vi "Auto Configuration.vi"() -> ()   [LabVIEW 2017]
uses:
  2018_Trobots_5013_Robot/Support Code/Blocks.ctl
  2018_Trobots_5013_Robot/Support Code/Routines.ctl
  2018_Trobots_5013_Robot/Auto Code/Block Clusters/Far--L.ctl
  2018_Trobots_5013_Robot/Auto Code/Block Clusters/end Sw--sq C1.ctl
  2018_Trobots_5013_Robot/Auto Code/Block Clusters/end cube--C1.ctl
  2018_Trobots_5013_Robot/Auto Code/Block Clusters/C1--d Hi.ctl
  2018_Trobots_5013_Robot/Auto Code/Block Clusters/C1--C3.ctl
  2018_Trobots_5013_Robot/Auto Code/Block Clusters/C3--C4.ctl
  2018_Trobots_5013_Robot/Auto Code/Block Clusters/d Hi--C1.ctl
  2018_Trobots_5013_Robot/Auto Code/Block Clusters/C3--End Sw.ctl
  2018_Trobots_5013_Robot/Auto Code/Block Clusters/C3--cube Sw.ctl
  2018_Trobots_5013_Robot/Auto Code/Block Clusters/M--front RSw.ctl
  2018_Trobots_5013_Robot/Auto Code/Block Clusters/L--C1.ctl
  2018_Trobots_5013_Robot/Auto Code/Block Clusters/C1--end cube.ctl
  2018_Trobots_5013_Robot/Auto Code/Block Clusters/L--end Sw.ctl
  2018_Trobots_5013_Robot/Auto Code/Block Clusters/front Sw--L.ctl
  2018_Trobots_5013_Robot/Auto Code/Block Clusters/M--front LSw.ctl
  2018_Trobots_5013_Robot/Auto Code/Block Clusters/SQ Hi--C1.ctl
  2018_Trobots_5013_Robot/Auto Code/Block Clusters/C1--sq Hi.ctl
  2018_Trobots_5013_Robot/Auto Code/Block Clusters/front Sw--P cube1.ctl
  2018_Trobots_5013_Robot/Auto Code/Block Clusters/P cube1--front Sw.ctl
  Routines and Block Data.ctl
  <vilib>/Rock Robotics/Network Tables/NT Write Boolean.vi
panel:
  in  "Reposition":bool
  out "appended path":path=path "C:/Program Files (x86)/FRC Dashboard/data/C1--end cube.jpg"
  out "Tab Control":T1(tab)=enum."2"
  in  "Far--L":T2={"1a"=0.0, "1d"=100.5, "1s"=0.8}
  in  "L--end Sw":T3={"1d"=48.0, "1s"=0.8, "2t"=3.0, "3a"=90.0, "4d"=21.5, "4s"=0.8}
  in  "end Sw--sq C1":T4={"1a"=-90.0, "1d"=-48.0, "1s"=-0.65, "2d"=67.25, "2s"=0.75}
  in  "end cube--C1":T5={"1a"=124.0, "1d"=0.0, "1s"=0.0, "2a"=0.0}
  in  "C1--d Hi":T6={"1t"=6.5, "2d"=55.0, "2s"=0.65, "3a"=38.0, "4d"=10.0, "4s"=0.5}
  in  "C1--C3":T7={"1a"=90.0, "2d"=185.0, "2s"=1.0}
  in  "C3 to C4":T8
  in  "d Hi--C1":T9={"1a"=38.0, "1d"=18.0, "1s"=0.8, "3t"=0.0, "4d"=33.0, "4s"=1.0}
  in  "C3--End Sw":T10={"1a"=90.0, "1d"=45.31, "1s"=0.8, "2a"=180.0, "3t"=3.0, "4d"=67.25, "4s"=0.7, "5a"=-90.0, "6d"=19.31, "6s"=0.5}
  in  "C3--cube Sw":T11
  in  "M--front LSw":T12={"1d"=14.0, "1s"=1.0, "2a"=-51.5, "3t"=3.0, "4d"=141.0, "4s"=1.0, "5a"=0.0, "6d"=19.5, "6s"=0.5}
  in  "M--front RSw":T13
  in  "front Sw--L":T14={"1d"=14.0, "1s"=-1.0, "2a"=90.0, "3t"=0.0, "4d"=58.25, "4s"=1.0, "5a"=0.0}
  in  "L--C1":T15={"1a"=0.0, "1d"=115.25, "1s"=0.8}
  in  "C1--end cube":T16={"1a"=124.0, "2d"=28.0, "2s"=0.65, "3g"=10.0, "4t"=1.0}
  in  "sq Hi--C1":T17
  in  "C1--sq Hi":T18
  in  "front Sw--P cube1":T19
  in  "P cube1--front Sw":T20={"1a"=0.0, "1d"=40.0, "1s"=-0.85, "2a"=-90.0, "1t"=3.0, "2d"=57.0, "2s"=1.0, "3d"=81.0, "3s"=0.65}
  in  "Remove":bool
  in  "Index":i32=1 min=1 step=1
  in  "Insert":bool
  in  "Routines":T21
  in  "Routine Blocks":T22[](array[typedef])=[enum."M--front LSw", enum."front Sw--L", enum."L--C1", enum."C1--end cube", enum."end cube--C1", enum."C1--d Hi", enum."", enum."", enum."", enum."", enum."", enum."", enum."", enum."", enum."", enum."", enum."", enum."", enum."", enum."", enum."", enum."", enum."", enum."", enum."", enum."", enum.""]
  in  "Cancel":bool
  in  "Done":bool
  in  "Block to Modify":T22=enum."Far--L"
  out "block picture":picture
  # "1"
  # "2"
  # "3"
  # "4"
  # "5"
  # "6"
  # "7"
  # "8"
  # "9"
  # "10"
  # "11"
  # "12"
  # "13"
  # "14"
  # "15"
  # "16"
  # "17"
  # "18"
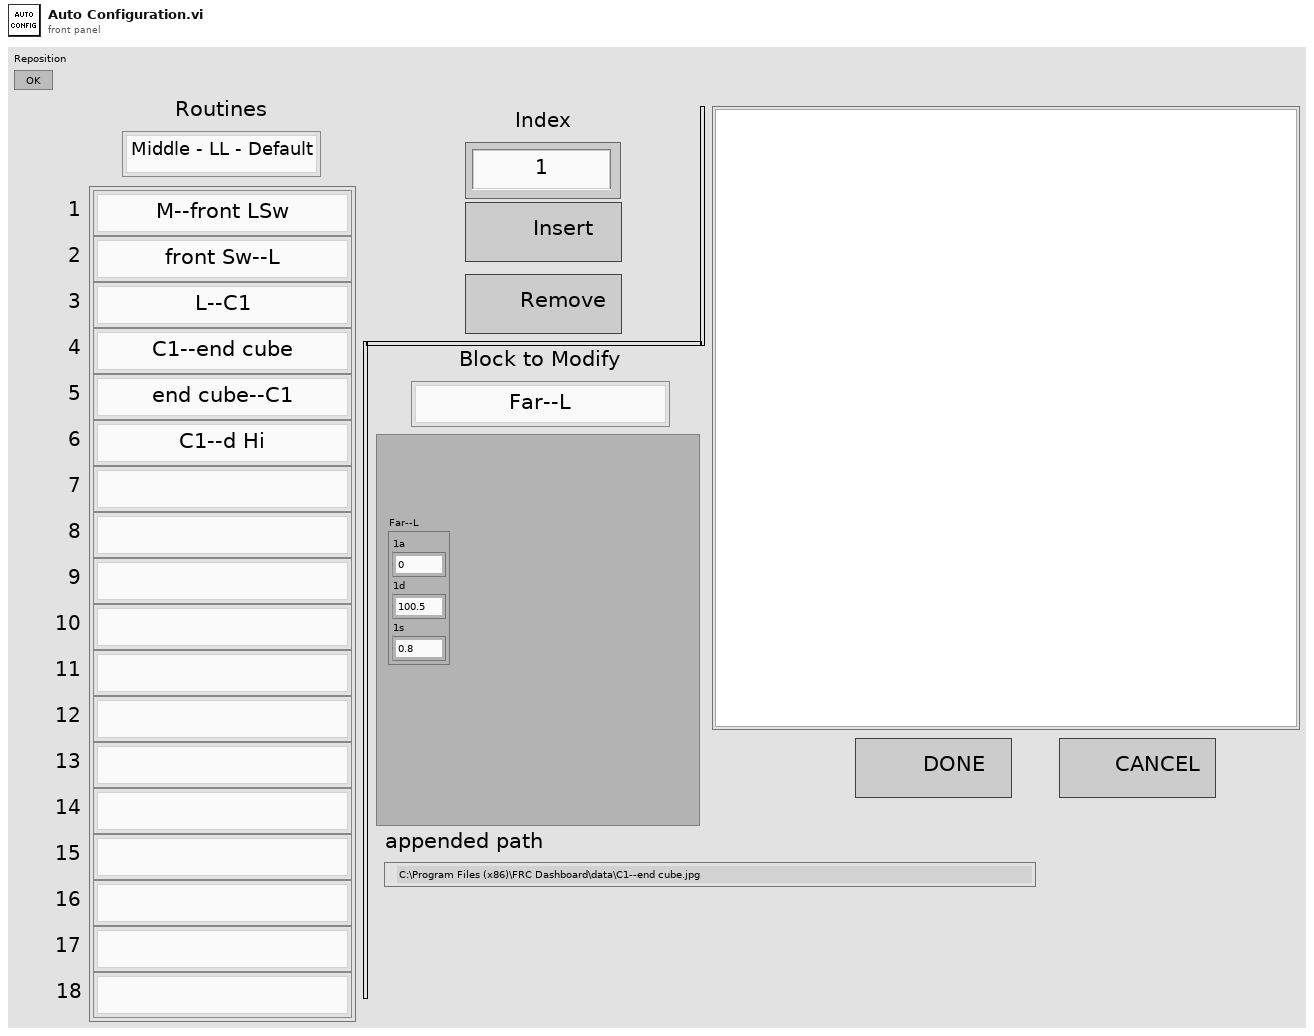
[diagram p1: front panel]
types:
  T1 = enum32{"0", "1", "2", "3", "4", "5", "6", "7", "8", "9", "9 2", "9 3", "9 4", "9 5", "front Sw--L", "L--C1", "C1--end cube", "C1--end cube 2", "C1--end cube 3", "C1--end cube 4", "C1--end cube 5"}
  T2 = typedef "Far--L.ctl" = cluster{"1a":dbl, "1d":dbl, "1s":dbl}
  T3 = typedef "L--end Sw.ctl" = cluster{"1d":dbl, "1s":dbl, "2t":dbl, "3a":dbl, "4d":dbl, "4s":dbl}
  T4 = typedef "end Sw--sq C1.ctl" = cluster{"1a":dbl, "1d":dbl, "1s":dbl, "2d":dbl, "2s":dbl}
  T5 = typedef "end cube--C1.ctl" = cluster{"1a":dbl, "1d":dbl, "1s":dbl, "2a":dbl}
  T6 = typedef "C1--d Hi.ctl" = cluster{"1t":dbl, "2d":dbl, "2s":dbl, "3a":dbl, "4d":dbl, "4s":dbl}
  T7 = typedef "C1--C3.ctl" = cluster{"1a":dbl, "2d":dbl, "2s":dbl}
  T8 = typedef "C3--C4.ctl" = cluster{"1a":dbl, "1d":dbl, "1s":dbl}
  T9 = typedef "d Hi--C1.ctl" = cluster{"1a":dbl, "1d":dbl, "1s":dbl, "3t":dbl, "4d":dbl, "4s":dbl}
  T10 = typedef "C3--End Sw.ctl" = cluster{"1a":dbl, "1d":dbl, "1s":dbl, "2a":dbl, "3t":dbl, "4d":dbl, "4s":dbl, "5a":dbl, "6d":dbl, "6s":dbl}
  T11 = typedef "C3--cube Sw.ctl" = cluster{"1a":dbl, "1d":dbl, "1s":dbl, "2a":dbl, "4d":dbl, "4s":dbl, "5t":dbl}
  T12 = typedef "M--front LSw.ctl" = cluster{"1d":dbl, "1s":dbl, "2a":dbl, "3t":dbl, "4d":dbl, "4s":dbl, "5a":dbl, "6d":dbl, "6s":dbl}
  T13 = typedef "M--front RSw.ctl" = cluster{"1a":dbl, "1d":dbl, "1s":dbl}
  T14 = typedef "front Sw--L.ctl" = cluster{"1d":dbl, "1s":dbl, "2a":dbl, "3t":dbl, "4d":dbl, "4s":dbl, "5a":dbl}
  T15 = typedef "L--C1.ctl" = cluster{"1a":dbl, "1d":dbl, "1s":dbl}
  T16 = typedef "C1--end cube.ctl" = cluster{"1a":dbl, "2d":dbl, "2s":dbl, "3g":dbl, "4t":dbl}
  T17 = typedef "SQ Hi--C1.ctl" = cluster{"1a":dbl, "1d":dbl, "1s":dbl, "2d":dbl, "2s":dbl}
  T18 = typedef "C1--sq Hi.ctl" = cluster{"1d":dbl, "1s":dbl, "2a":dbl, "2d":dbl, "2s":dbl}
  T19 = typedef "front Sw--P cube1.ctl" = cluster{"1a":dbl, "1d":dbl, "1s":dbl, "2a":dbl, "2d":dbl, "2s":dbl, "3d":dbl, "3s":dbl, "1t":dbl}
  T20 = typedef "P cube1--front Sw.ctl" = cluster{"1a":dbl, "1d":dbl, "1s":dbl, "2a":dbl, "1t":dbl, "2d":dbl, "2s":dbl, "3d":dbl, "3s":dbl}
  T21 = typedef "Routines.ctl" = enum16{"Middle - LL - Default", "Middle - LR - Default", "Middle - RL - Default", "Middle - RR - Default", "Far Right - LL - Default", "Far Right - LR - Default", "Far Right - RL - Default", "Far Right - RR - Default", "Far Left - LL - Default", "Far Left - LR - Default", "Far Left - RL - Default", "Far Left - RR - Default", "Middle - LL - Scale", "Middle - LR - Scale", "Middle - RL - Scale", "Middle - RR - Scale", "Far Right - LL - Scale", "Far Right - LR - Scale", "Far Right - RL - Scale", "Far Right - RR - Scale", "Far Left - LL - Scale", "Far Left - LR - Scale", "Far Left - RL - Scale", "Far Left - RR - Scale", "Middle - LL - Switch", "Middle - LR - Switch", "Middle - RL - Switch", "Middle - RR - Switch", "Far Right - LL - Switch", "Far Right - LR - Switch", "Far Right - RL - Switch", "Far Right - RR - Switch", "Far Left - LL - Switch", "Far Left - LR - Switch", "Far Left - RL - Switch", "Far Left - RR - Switch"}
  T22 = typedef "Blocks.ctl" = enum16{"", "Wait 1s", "Far--L", "L--end Sw", "end Sw--sq C1", "end cube--C1", "C1--d Hi", "C1--C3", "C3--C4", "d Hi--C1", "C3--end Sw", "C3--cube Sw", "M--front LSw", "M--front RSw", "front Sw--L", "L--C1", "C1--end cube", "sq Hi--C1", "C1--sq Hi", "front Sw--P cube1", "P cube1--front Sw"}
  T23 = typedef "Routines and Block Data.ctl" = cluster{"Routines":T22[][], "Block Data Array":variant[]}
  T24 = typedef "imagedata.ctl" = cluster{"image type":i32, "image depth":i32, "image":u8[], "mask":u8[], "colors":u32[], "Rectangle":cluster{"left":i16, "top":i16, "right":i16, "bottom":i16}}
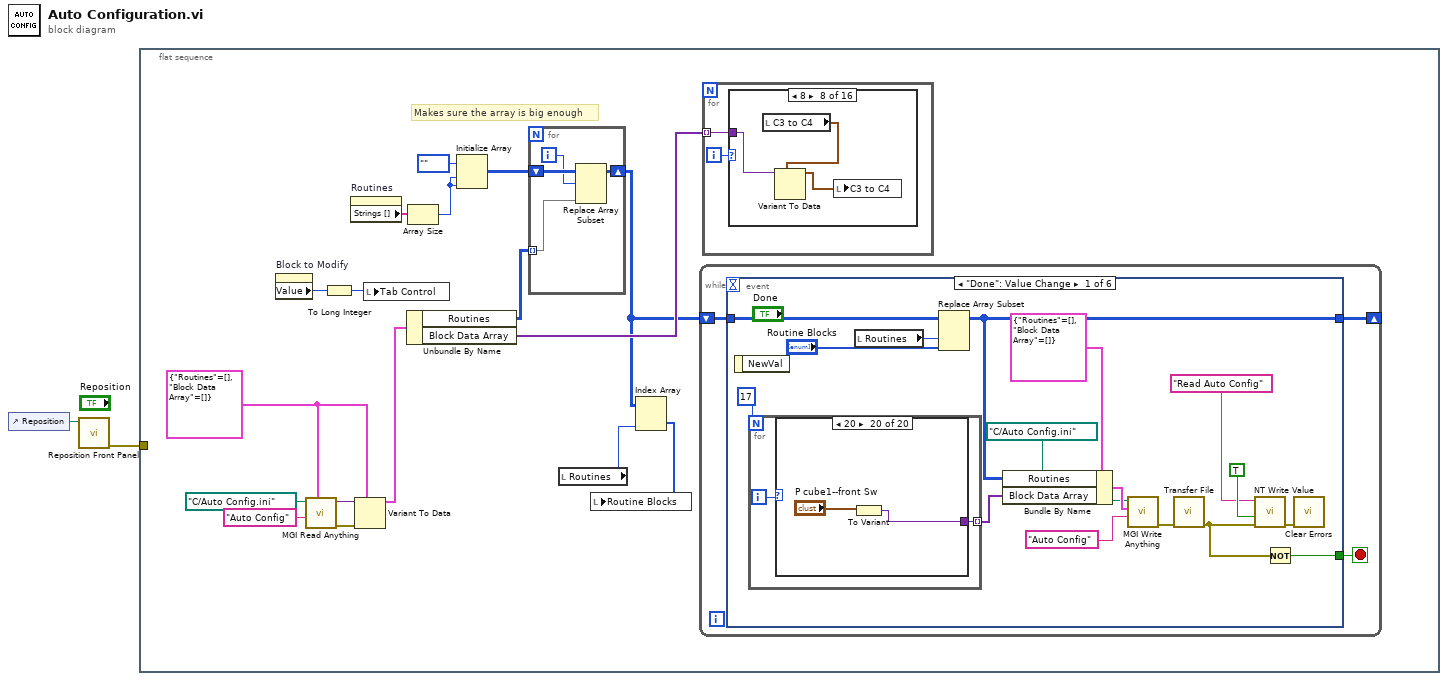
[diagram p0: block diagram]
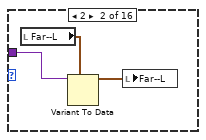
[diagram p3: hidden frame]
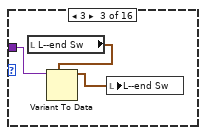
[diagram p4: hidden frame]
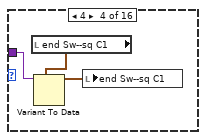
[diagram p5: hidden frame]
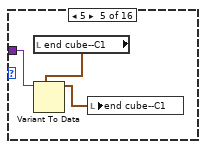
[diagram p6: hidden frame]
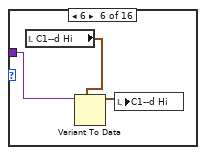
[diagram p7: hidden frame]
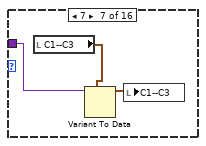
[diagram p8: hidden frame]
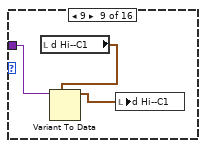
[diagram p9: hidden frame]
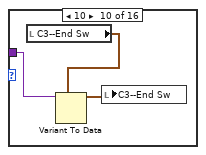
[diagram p10: hidden frame]
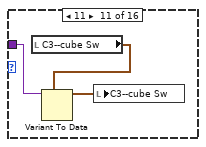
[diagram p11: hidden frame]
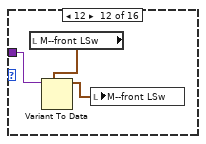
[diagram p12: hidden frame]
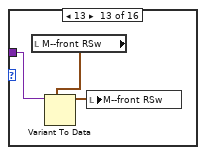
[diagram p13: hidden frame]
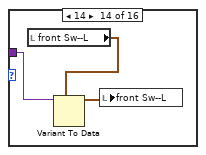
[diagram p14: hidden frame]
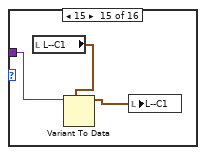
[diagram p15: hidden frame]
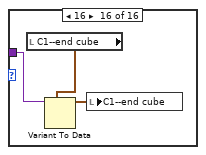
[diagram p16: hidden frame]
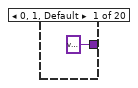
[diagram p17: hidden frame]
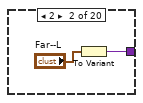
[diagram p18: hidden frame]
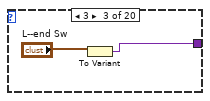
[diagram p19: hidden frame]
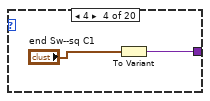
[diagram p20: hidden frame]
diagram:
  n1 = control-ref of="Reposition"() -> (w1:refnum<vi>)
  n2 = call "Reposition Front Panel.vi"("reference"=w1) -> ("error out"=w2:errorcluster)  [unwired: 10 in]
  n3 = flat-sequence {
    tunnel: w2 -> [_]
    frame #0 {
      w15 = T23 {"Routines"=[], "Block Data Array"=[]} ("Routines and Block Data")
      # "Makes sure the array is big enough"
      n4 = property on="Block to Modify" class="Enum (strict)"() -> ("Value"=w11:T22)  [unwired: 2 in, 2 out]
      n5 = call <userlib>:"MGI Read Anything.vi"("Type of Anything"=w15, "Section Name (Name of \"Type of Anything\")"="Auto Config" ("Section Name (Name of \"Type of Anything\")"), "Path (dialog)"=path "C:/Auto Config.ini") -> ("Error Out"=w19:errorcluster, "Anything"=w18:variant)  [unwired: 5 in, 2 out]
      n6 = To Long Integer(number=w11) -> (32bit integer=w10:i32)
      n7 = property on="Routines" class="Enum (strict)"() -> ("Strings []"=w6:string[])  [unwired: 2 in, 2 out]
      n8 = Variant To Data(error in=w19, type=w15, Variant=w18) -> (data=w16:T23)  [unwired: 1 out]
      n9 = local write "Tab Control"(w10) -> ()
      n10 = Unbundle By Name(w16) -> ("Routines"=w4:T22[][], "Block Data Array"=w9:variant[])
      n11 = Array Size(array=w6) -> (size(s)=w5:i32)
      n12 = Initialize Array(Blocks."" ("Blocks"), w5, w5) -> (w7:T22[][])
      n13 = for {
        tunnel: w4 -> [w168] mode=indexing
        shift-right: [w166] -> w3
        shift-left: w7 -> [w169]
        i -> [w167]
        n14 = Replace Array Subset(array=w169, new element=w168, index (row)=w167) -> (w166:T22[][])  [unwired: 1 in]
      }
      n15 = local read "Routines"() -> (w13:T21)
      n16 = Index Array(array=w3, index (col)=w13) -> (element=w12:T22[])  [unwired: 1 in]
      n17 = local write "Routine Blocks"(w12) -> ()
      n18 = while {
        shift-right: [w67] -> _
        shift-left: w3 -> [w68]
        stop <- w69 stop-if-true
        n19 = event shown="[0] \"Done\": Value Change" {
          selector: _ -> [_ _ _ _ _ _]
          dyn-events: _ -> [_ _ _ _ _ _]
          timeout: _ -> [_ _ _ _ _ _]
          tunnel: [w70 TRUE _ _ _ _] -> w69
          tunnel: w68 -> [w85 w127 w134 w146 w159 w164]
          tunnel: [w80 w127 w134 w145 w154 w161] -> w67
          event "Done": Value Change {
            n20 = event-data() -> ()  [unwired: 1 in, 1 out]
            n21 = for {
              N: 17 -> [_]
              tunnel: [w87] -> w72 mode=indexing
              i -> [w86]
              n22 = case shown="20" w86 {
                tunnel: [variant ("Variant") w90 w92 w94 w95 w97 w99 w101 w103 w105 w107 w110 w111 w114 w115 w117 w119 w121 w123 w125] -> w87
                frame 0, 1, Default {
                }
                frame 2 {
                  n23 = To Variant(anything="Far--L") -> (Variant=w90:variant)
                }
                frame 3 {
                  n24 = To Variant(anything="L--end Sw") -> (Variant=w92:variant)
                }
                frame 4 {
                  n25 = To Variant(anything="end Sw--sq C1") -> (Variant=w94:variant)
                }
                frame 5 {
                  n26 = To Variant(anything="end cube--C1") -> (Variant=w95:variant)
                }
                frame 6 {
                  n27 = To Variant(anything="C1--d Hi") -> (Variant=w97:variant)
                }
                frame 7 {
                  n28 = To Variant(anything="C1--C3") -> (Variant=w99:variant)
                }
                frame 8 {
                  n29 = To Variant(anything="C3 to C4") -> (Variant=w101:variant)
                }
                frame 9 {
                  n30 = To Variant(anything="d Hi--C1") -> (Variant=w103:variant)
                }
                frame 10 {
                  n31 = To Variant(anything="C3--End Sw") -> (Variant=w105:variant)
                }
                frame 11 {
                  n32 = To Variant(anything="C3--cube Sw") -> (Variant=w107:variant)
                }
                frame 12 {
                  n33 = To Variant(anything="M--front LSw") -> (Variant=w110:variant)
                }
                frame 13 {
                  n34 = To Variant(anything="M--front RSw") -> (Variant=w111:variant)
                }
                frame 14 {
                  n35 = To Variant(anything="front Sw--L") -> (Variant=w114:variant)
                }
                frame 15 {
                  n36 = To Variant(anything="L--C1") -> (Variant=w115:variant)
                }
                frame 16 {
                  n37 = To Variant(anything="C1--end cube") -> (Variant=w117:variant)
                }
                frame 17 {
                  n38 = To Variant(anything="sq Hi--C1") -> (Variant=w119:variant)
                }
                frame 18 {
                  n39 = To Variant(anything="front Sw--P cube1") -> (Variant=w121:variant)
                }
                frame 19 {
                  n40 = To Variant(anything="C1--sq Hi") -> (Variant=w123:variant)
                }
                frame 20 {
                  n41 = To Variant(anything="P cube1--front Sw") -> (Variant=w125:variant)
                }
              }
            }
            n42 = local read "Routines"() -> (w75:T21)
            n43 = Replace Array Subset(array=w85, new element="Routine Blocks", index (col)=w75) -> (w80:T22[][])  [unwired: 1 in]
            n44 = Bundle By Name(cluster=T23 {"Routines"=[], "Block Data Array"=[]} ("Routines and Block Data"), "Routines"=w80, "Block Data Array"=w72) -> (w82:T23)
            n45 = call <userlib>:"MGI Write Anything.vi"("Section Name (Name of \"Anything\")"="Auto Config" ("Section Name (Name of \"Anything\")"), "Anything"=w82, "Path (dialog)"=path "C:/Auto Config.ini") -> ("Error Out"=w76:errorcluster)  [unwired: 6 in, 2 out]
            n46 = call "Transfer File.vi"("error in (no error)"=w76) -> ("error out"=w71:errorcluster)  [unwired: 10 in]
            n47 = call-poly <vilib>:"NT Write Value.vi"("error in"=w71, "Boolean"=TRUE, "Name"="Read Auto Config") -> ("error out"=w74:errorcluster)  [unwired: 8 in]
            n48 = Not(x=w71) -> (.not. x?=w70:bool)
            n49 = call <vilib>:"Clear Errors.vi"("error in (no error)"=w74) -> ()  [unwired: 5 in, 2 out]
          }
          event "Cancel": Value Change {
            n50 = event-data() -> ()  [unwired: 1 in, 1 out]
          }
          event Value Change {
            n51 = event-data() -> ()  [unwired: 1 in, 1 out]
            n52 = property on="Block to Modify" class="Enum (strict)"() -> ("Value"=w133:T22)  [unwired: 2 in, 2 out]
            n53 = Format Into String(format string="%s", "Block to Modify") -> (resulting string=w140:string)  [unwired: 2 in, 1 out]
            n54 = To Long Integer(number=w133) -> (32bit integer=→"Tab Control":i32)
            n55 = Concatenate Strings(w140, ".jpg" ("string")) -> (w138:string)
            n56 = Build Path(base path=path "C:/Program Files (x86)/FRC Dashboard/data" ("Path (dialog)"), name or relative path=w138) -> (appended path=w135:path)
            "appended path" <- w135
            n57 = call <vilib>:"Read JPEG File.vi"("path to JPEG file"=w135) -> ("error out"=w130:errorcluster, "image data"=w136:T24)  [unwired: 8 in, 1 out]
            n58 = call <vilib>:"Draw Flattened Pixmap.vi"("image data"=w136) -> ("new picture"=→"block picture":picture)  [unwired: 8 in]
            n59 = call <vilib>:"Clear Errors.vi"("error in (no error)"=w130) -> ()  [unwired: 5 in, 2 out]
          }
          event "Insert": Value Change {
            n60 = event-data() -> ()  [unwired: 1 in, 2 out]
            n61 = local read "Routine Blocks"() -> (w142:T22[])
            n62 = Decrement(x="Index") -> (x-1=w148:i32)
            n63 = local read "Routines"() -> (w144:T21)
            n64 = Insert Into Array(array=w142, index=w148, new element=Blocks."" ("new element/subarray")) -> (w143:T22[])
            n65 = local write "Routine Blocks"(w143) -> ()
            n66 = Replace Array Subset(array=w146, new element=w143, index (col)=w144) -> (w145:T22[][])  [unwired: 1 in]
          }
          event "Remove": Value Change {
            # "take everything below the index in that routine\nand move it all up 1 spot in the array"
            n67 = event-data() -> ()  [unwired: 1 in, 2 out]
            n68 = local read "Index"() -> (w157:i32)
            n69 = local read "Routine Blocks"() -> (w150:T22[])
            n70 = Decrement(x=w157) -> (x-1=w156:i32)
            n71 = Array Subset(array=w150, index=w157) -> (w158:T22[])  [unwired: 1 in]
            n72 = Build Array (concatenate)(w158, Blocks."" ("Blocks")) -> (w153:T22[])
            n73 = local read "Routines"() -> (w155:T21)
            n74 = Replace Array Subset(array=w150, new element=w153, index=w156) -> (w151:T22[])
            n75 = Replace Array Subset(array=w159, new element=w151, index (col)=w155) -> (w154:T22[][])  [unwired: 1 in]
            n76 = local write "Routine Blocks"(w151) -> ()
          }
          event Value Change {
            n77 = event-data() -> ("OldVal"=w162:T21)  [unwired: 1 in]
            n78 = local read "Routine Blocks"() -> (w163:T22[])
            n79 = Replace Array Subset(array=w164, new element=w163, index (col)=w162) -> (w161:T22[][])  [unwired: 1 in]
            n80 = Index Array(array=w161, index (col)="Routines") -> (element=w165:T22[])  [unwired: 1 in]
            n81 = local write "Routine Blocks"(w165) -> ()
          }
        }
      }
      n82 = for {
        tunnel: w9 -> [w20] mode=indexing
        i -> [w21]
        n83 = case shown="8" w21 {
          tunnel: w20 -> [_ w24 w27 w30 w33 w34 w37 w42 w45 w46 w49 w54 w56 w58 w63 w65]
          frame 0, Default {
          }
          frame 2 {
            n84 = local read "Far--L"() -> (w23:T2)
            n85 = Variant To Data(type=w23, Variant=w24) -> (data=w22:T2)  [unwired: 1 in, 1 out]
            n86 = local write "Far--L"(w22) -> ()
          }
          frame 3 {
            n87 = local read "L--end Sw"() -> (w26:T3)
            n88 = Variant To Data(type=w26, Variant=w27) -> (data=w25:T3)  [unwired: 1 in, 1 out]
            n89 = local write "L--end Sw"(w25) -> ()
          }
          frame 4 {
            n90 = local read "end Sw--sq C1"() -> (w29:T4)
            n91 = Variant To Data(type=w29, Variant=w30) -> (data=w28:T4)  [unwired: 1 in, 1 out]
            n92 = local write "end Sw--sq C1"(w28) -> ()
          }
          frame 5 {
            n93 = local read "end cube--C1"() -> (w32:T5)
            n94 = Variant To Data(type=w32, Variant=w33) -> (data=w31:T5)  [unwired: 1 in, 1 out]
            n95 = local write "end cube--C1"(w31) -> ()
          }
          frame 6 {
            n96 = local read "C1--d Hi"() -> (w35:T6)
            n97 = Variant To Data(type=w35, Variant=w34) -> (data=w36:T6)  [unwired: 1 in, 1 out]
            n98 = local write "C1--d Hi"(w36) -> ()
          }
          frame 7 {
            n99 = local read "C1--C3"() -> (w38:T7)
            n100 = Variant To Data(type=w38, Variant=w37) -> (data=w39:T7)  [unwired: 1 in, 1 out]
            n101 = local write "C1--C3"(w39) -> ()
          }
          frame 8 {
            n102 = local read "C3 to C4"() -> (w41:T8)
            n103 = Variant To Data(type=w41, Variant=w42) -> (data=w40:T8)  [unwired: 1 in, 1 out]
            n104 = local write "C3 to C4"(w40) -> ()
          }
          frame 9 {
            n105 = local read "d Hi--C1"() -> (w44:T9)
            n106 = Variant To Data(type=w44, Variant=w45) -> (data=w43:T9)  [unwired: 1 in, 1 out]
            n107 = local write "d Hi--C1"(w43) -> ()
          }
          frame 10 {
            n108 = local read "C3--End Sw"() -> (w48:T10)
            n109 = Variant To Data(type=w48, Variant=w46) -> (data=w47:T10)  [unwired: 1 in, 1 out]
            n110 = local write "C3--End Sw"(w47) -> ()
          }
          frame 11 {
            n111 = local read "C3--cube Sw"() -> (w50:T11)
            n112 = Variant To Data(type=w50, Variant=w49) -> (data=w51:T11)  [unwired: 1 in, 1 out]
            n113 = local write "C3--cube Sw"(w51) -> ()
          }
          frame 12 {
            n114 = local read "M--front LSw"() -> (w53:T12)
            n115 = Variant To Data(type=w53, Variant=w54) -> (data=w52:T12)  [unwired: 1 in, 1 out]
            n116 = local write "M--front LSw"(w52) -> ()
          }
          frame 13 {
            n117 = local read "M--front RSw"() -> (w55:T13)
            n118 = Variant To Data(type=w55, Variant=w56) -> (data=w57:T13)  [unwired: 1 in, 1 out]
            n119 = local write "M--front RSw"(w57) -> ()
          }
          frame 14 {
            n120 = local read "front Sw--L"() -> (w59:T14)
            n121 = Variant To Data(type=w59, Variant=w58) -> (data=w60:T14)  [unwired: 1 in, 1 out]
            n122 = local write "front Sw--L"(w60) -> ()
          }
          frame 15 {
            n123 = local read "L--C1"() -> (w62:T15)
            n124 = Variant To Data(type=w62, Variant=w63) -> (data=w61:T15)  [unwired: 1 in, 1 out]
            n125 = local write "L--C1"(w61) -> ()
          }
          frame 16 {
            n126 = local read "C1--end cube"() -> (w64:T16)
            n127 = Variant To Data(type=w64, Variant=w65) -> (data=w66:T16)  [unwired: 1 in, 1 out]
            n128 = local write "C1--end cube"(w66) -> ()
          }
        }
      }
    }
  }
